vi "NMRvme3.vi"() -> ()   [LabVIEW 2013]
uses:
  <vilib>/Utility/file.llb/Read From Spreadsheet File (DBL).vi
  <vilib>/Analysis/NI_AALBase.lvlib
panel:
  in  "RemovePed":bool=TRUE
  in  "IF / LOG Det":bool
  in  "Q curve file":string="realback213.txt"
  out "File name 2":string="C:\\users\\plm\\Desktop\\rssmt\\realback213.txt"
  in  "AutoBaseline":bool
  out "RF OK":bool=TRUE
  out "Peak area (V-MHz)":sgl=0.007902089 format="%.3f"
  in  "Gauss Fit":bool
  out "NMR Graph + Fit":cluster{cluster{dbl, "Numeric":dbl}[]}[](graph)=[{[{224.37, "Numeric"=0.011213333333333334}, {224.372, "Numeric"=0.009013333333333333}, {224.374, "Numeric"=0.006013333333333334}, {224.376, "Numeric"=0.005013333333333333}, {224.37800000000001, "Numeric"=0.0029133333333333333}, {224.38, "Numeric"=-0.002886666666666667}, {224.382, "Numeric"=0.0015133333333333331}, {224.38400000000001, "Numeric"=0.006213333333333333}, {224.386, "Numeric"=-0.000986666666666667}, {224.388, "Numeric"=-0.009586666666666667}, {224.39000000000001, "Numeric"=-0.007886666666666667}, {224.392, "Numeric"=-0.0054866666666666675}, {224.394, "Numeric"=-0.011186666666666666}, {224.39600000000002, "Numeric"=-0.005086666666666666}, {224.398, "Numeric"=0.003413333333333333}, {224.4, "Numeric"=-0.006986666666666667}, {224.40200000000002, "Numeric"=-0.013286666666666667}, {224.404, "Numeric"=-0.003986666666666667}, {224.406, "Numeric"=0.003513333333333333}, {224.40800000000002, "Numeric"=-0.010286666666666666}, {224.41, "Numeric"=-0.012286666666666666}, {224.412, "Numeric"=-0.002686666666666667}, {224.41400000000002, "Numeric"=-0.0074866666666666675}, {224.416, "Numeric"=-0.013786666666666666}, {224.418, "Numeric"=-0.008786666666666667}, {224.42000000000002, "Numeric"=-0.001286666666666667}, {224.422, "Numeric"=-0.004586666666666667}, {224.424, "Numeric"=-0.013886666666666667}, {224.426, "Numeric"=-0.007186666666666668}, {224.428, "Numeric"=-0.001986666666666667}, {224.43, "Numeric"=-0.006186666666666667}, {224.432, "Numeric"=-0.002586666666666667}, {224.434, "Numeric"=0.006213333333333333}, {224.436, "Numeric"=0.006313333333333334}, {224.438, "Numeric"=0.003913333333333333}, {224.44, "Numeric"=0.009913333333333333}, {224.442, "Numeric"=0.020313333333333333}, {224.444, "Numeric"=0.018113333333333332}, {224.446, "Numeric"=0.02461333333333333}, {224.448, "Numeric"=0.038213333333333335}, {224.45, "Numeric"=0.048113333333333334}, {224.452, "Numeric"=0.059713333333333334}, {224.454, "Numeric"=0.07631333333333333}, {224.456, "Numeric"=0.11191333333333334}, {224.458, "Numeric"=0.14051333333333332}, {224.46, "Numeric"=0.17031333333333334}, {224.462, "Numeric"=0.22211333333333333}, {224.464, "Numeric"=0.2830133333333333}, {224.466, "Numeric"=0.3263133333333333}, {224.468, "Numeric"=0.3479133333333333}, {224.47, "Numeric"=0.36471333333333333}, {224.472, "Numeric"=0.3424133333333333}, {224.474, "Numeric"=0.2951133333333333}, {224.476, "Numeric"=0.23841333333333334}, {224.478, "Numeric"=0.20081333333333334}, {224.48, "Numeric"=0.16211333333333333}, {224.482, "Numeric"=0.12461333333333333}, {224.484, "Numeric"=0.09951333333333333}, {224.486, "Numeric"=0.09201333333333334}, {224.488, "Numeric"=0.07011333333333333}, {224.49, "Numeric"=0.05211333333333334}, {224.492, "Numeric"=0.04461333333333334}, {224.494, "Numeric"=0.04271333333333333}, {224.496, "Numeric"=0.02851333333333333}, {224.498, "Numeric"=0.020213333333333333}, {224.5, "Numeric"=0.023113333333333333}, {224.502, "Numeric"=0.02411333333333333}, {224.504, "Numeric"=0.009413333333333334}, {224.506, "Numeric"=0.010313333333333334}, {224.508, "Numeric"=0.016413333333333332}, {224.51, "Numeric"=0.007913333333333333}, {224.512, "Numeric"=-0.005086666666666666}, {224.514, "Numeric"=-0.001386666666666667}, {224.516, "Numeric"=0.008913333333333334}, {224.518, "Numeric"=0.006013333333333334}, {224.51999999999998, "Numeric"=-0.00048666666666666693}, {224.522, "Numeric"=-0.000986666666666667}, {224.524, "Numeric"=0.0006133333333333329}, {224.52599999999998, "Numeric"=-0.001286666666666667}, {224.528, "Numeric"=0.001813333333333333}, {224.53, "Numeric"=0.011613333333333333}, {224.53199999999998, "Numeric"=0.002213333333333333}, {224.534, "Numeric"=-0.002686666666666667}, {224.536, "Numeric"=0.006913333333333334}, {224.53799999999998, "Numeric"=0.005213333333333334}, {224.54, "Numeric"=-8.666666666666718e-05}, {224.542, "Numeric"=-0.000186666666666667}, {224.54399999999998, "Numeric"=0.0017133333333333328}, {224.546, "Numeric"=0.0026133333333333334}, {224.548, "Numeric"=-0.002786666666666667}, {224.54999999999998, "Numeric"=0.004013333333333332}, {224.552, "Numeric"=0.016813333333333333}, {224.554, "Numeric"=0.004113333333333333}, {224.55599999999998, "Numeric"=-0.003086666666666667}, {224.558, "Numeric"=0.004413333333333333}, {224.56, "Numeric"=0.011913333333333333}, {224.56199999999998, "Numeric"=0.004713333333333333}, {224.564, "Numeric"=0.0029133333333333333}, {224.566, "Numeric"=0.012713333333333333}, {224.56799999999998, "Numeric"=0.011013333333333333}, {224.57, "Numeric"=0.0006133333333333329}]}]
  in  "Amp of Q curve":dbl=1.7999999999999998 min=0.0 max=3.0 step=0.01 format="%_3f"
  in  "Subtract Q curve":bool
  in  "Adjust Tune":bool
  out "Ped Offset":dbl(graph)=0.002486666666666667
  out "Pedestal Difference":dbl(graph)=0.006853333333333334
  out "# Good Spectra":i32=49
  in  "Quality cuts":bool=TRUE
  out "Pedestal OK":bool=TRUE
  out "Sweep #":i32=5
  out "1st Sweep":bool
  out "ADC volts OK":bool=TRUE
  out "Peak Height Distribution":cluster{"Y":dbl[], "Y":dbl[]}[](graph)=[{"Y"=[0.003398266666666667, 0.0034614666666666666, 0.0035246666666666664, 0.0035878666666666666, 0.0036510666666666664, 0.0037142666666666667, 0.0037774666666666665, 0.0038406666666666663, 0.0039038666666666665, 0.003967066666666666, 0.0040302666666666665, 0.004093466666666666, 0.004156666666666666, 0.004219866666666666, 0.004283066666666666, 0.004346266666666666, 0.004409466666666666, 0.004472666666666666, 0.004535866666666666, 0.004599066666666666, 0.004662266666666666, 0.004725466666666666, 0.004788666666666666, 0.004851866666666666, 0.0049150666666666655, 0.004978266666666666, 0.005041466666666666, 0.005104666666666665, 0.005167866666666666, 0.005231066666666666, 0.005294266666666665, 0.005357466666666665, 0.005420666666666666, 0.005483866666666665, 0.005547066666666665, 0.0056102666666666655, 0.005673466666666666, 0.005736666666666665, 0.005799866666666665, 0.0058630666666666656, 0.005926266666666665, 0.005989466666666665, 0.006052666666666665, 0.006115866666666665, 0.006179066666666665, 0.006242266666666665, 0.006305466666666665, 0.006368666666666665, 0.006431866666666665, 0.0064950666666666644, 0.006558266666666665, 0.006621466666666665, 0.006684666666666664, 0.0067478666666666645, 0.006811066666666665, 0.006874266666666665, 0.006937466666666664, 0.007000666666666665, 0.007063866666666665, 0.007127066666666664, 0.007190266666666664, 0.007253466666666665, 0.007316666666666664, 0.007379866666666664, 0.0074430666666666645, 0.007506266666666664, 0.007569466666666664, 0.007632666666666664, 0.007695866666666664, 0.007759066666666664, 0.007822266666666664, 0.007885466666666664, 0.007948666666666665, 0.008011866666666664, 0.008075066666666663, 0.008138266666666664, 0.008201466666666664, 0.008264666666666663, 0.008327866666666664, 0.008391066666666664, 0.008454266666666663, 0.008517466666666664, 0.008580666666666664, 0.008643866666666663, 0.008707066666666664, 0.008770266666666663, 0.008833466666666663, 0.008896666666666664, 0.008959866666666663, 0.009023066666666663, 0.009086266666666664, 0.009149466666666663, 0.009212666666666662, 0.009275866666666664, 0.009339066666666663, 0.009402266666666662, 0.009465466666666663, 0.009528666666666663, 0.009591866666666662, 0.009655066666666663], "Y"=[1.0, 0.0, 0.0, 0.0, 0.0, 0.0, 0.0, 0.0, 0.0, 1.0, 0.0, 2.0, 0.0, 1.0, 0.0, 0.0, 2.0, 0.0, 0.0, 0.0, 3.0, 2.0, 2.0, 1.0, 2.0, 0.0, 2.0, 0.0, 0.0, 2.0, 0.0, 0.0, 1.0, 1.0, 0.0, 0.0, 0.0, 0.0, 0.0, 0.0, 1.0, 1.0, 0.0, 1.0, 1.0, 0.0, 2.0, 0.0, 0.0, 0.0, 0.0, 0.0, 0.0, 0.0, 1.0, 1.0, 1.0, 0.0, 1.0, 0.0, 1.0, 0.0, 0.0, 0.0, 0.0, 0.0, 1.0, 2.0, 0.0, 2.0, 0.0, 0.0, 0.0, 0.0, 0.0, 0.0, 1.0, 1.0, 1.0, 0.0, 0.0, 0.0, 2.0, 0.0, 0.0, 1.0, 0.0, 0.0, 1.0, 0.0, 1.0, 1.0, 0.0, 0.0, 0.0, 0.0, 0.0, 0.0, 0.0, 1.0]}]
  in  "# of Sweeps":i32=50
  out "Std Dev (V)":dbl=0.001709574673437506 format="%_2g"
  out "Peak mean (V)":dbl=0.006236360544217688 format="%_4g"
  out "Peak Height":dbl(graph)=0.36471333333333333
  in  "Raw Data":bool=TRUE
  in  "Tank RF ON":bool=TRUE
  in  "IF Atten (dB)":i8 min=0 max=35 step=5
  in  "IFoffset (V)":dbl=-1.3469355999999992 min=-5.0 max=5.0 step=0.001 format="%.4f"
  in  "Tune  (V)":dbl=1.0946000000000007 min=0.0 max=5.0 step=0.001 format="%.4f"
  in  "Hi / Lo IF Gain":bool
  out "Voltage Array":sgl[](array[numeric])=[0.0137, 0.0115, 0.0085, 0.0075, 0.0054, -0.0004, 0.004, 0.0087, 0.0015, -0.0071, -0.0054, -0.003, -0.0087, -0.0026, 0.0059, -0.0045, -0.0108, -0.0015, 0.006, -0.0078, -0.0098, -0.0002, -0.005, -0.0113, -0.0063, 0.0012, -0.0021, -0.0114, -0.0047, 0.0005, -0.0037, -0.0001, 0.0087, 0.0088, 0.0064, 0.0124, 0.0228, 0.0206, 0.0271, 0.0407, 0.0506, 0.0622, 0.0788, 0.1144, 0.143, 0.1728, 0.2246, 0.2855, 0.3288, 0.3504, 0.3672, 0.3449, 0.2976, 0.2409, 0.2033, 0.1646, 0.1271, 0.102, 0.0945, 0.0726, 0.0546, 0.0471, 0.0452, 0.031, 0.0227, 0.0256, 0.0266, 0.0119, 0.0128, 0.0189, 0.0104, -0.0026, 0.0011, 0.0114, 0.0085, 0.002, 0.0015, 0.0031, 0.0012, 0.0043, 0.0141, 0.0047, -0.0002, 0.0094, 0.0077, 0.0024, 0.0023, 0.0042, 0.0051, -0.0003, 0.0065, 0.0193, 0.0066, -0.0006, 0.0069, 0.0144, 0.0072, 0.0054, 0.0152, 0.0135, 0.0031] format="%.4f"
  in  "Invert Polarity":bool
  out "Pedestal Diff (V)":sgl=0.006853333 format="%.3f"
  out "Peak amp (V)":sgl=0.36471334 format="%.3f"
  in  "Save Data to File":bool
  in  "RF Level (dBm)":dbl=-1.0 min=-10.0 max=1.0 step=0.1 format="%.2f"
  out "SMT error out":errorcluster
  out "Sample RMS (V)":dbl=0.01349207920792079 format="%.4f"
  in  "# Sample/step":i32=100 min=1 max=1000 step=100
  in  "ADC Rate (Hz)":i32=10000 min=1 max=20000 step=1000
  in  "ADC Range":i32(ring)=1 items=["+- 10 V"=1, "+- 2.5 V"=3]
  in  "Step Width (MHz)":dbl=0.002 min=0.0 max=1000.0 step=0.0005 format="%.4f"
  in  "Freq Span (MHz)":dbl=0.2 min=0.0 max=3000.0 step=0.1 format="%.3f"
  in  "Center Freq (MHz)":dbl=224.47 min=0.005 max=6000.0 step=0.1 format="%.3f"
  in  "Sweep Mode":u16(ring)=3 items=["Off", "Single", "Auto", "Step"]
  in  "GPIB Addr (28)":refnum<visa-resource-name>="GPIB0::28::INSTR"
  # "Settings"
  # "E1039 Prototype NMR Control Panel"
  # "D\nA\nC"
  # "R\nF\n\nG\ne\nn\ne\nr\na\nt\no\nr"
  # "A\nD\nC"
  # "D\na\nt\na"
  # "I\n/\nO"
  # "Results"
  # "A\nv\ne\nr\na\ng\ne"
  # "S\nw\ne\ne\np"
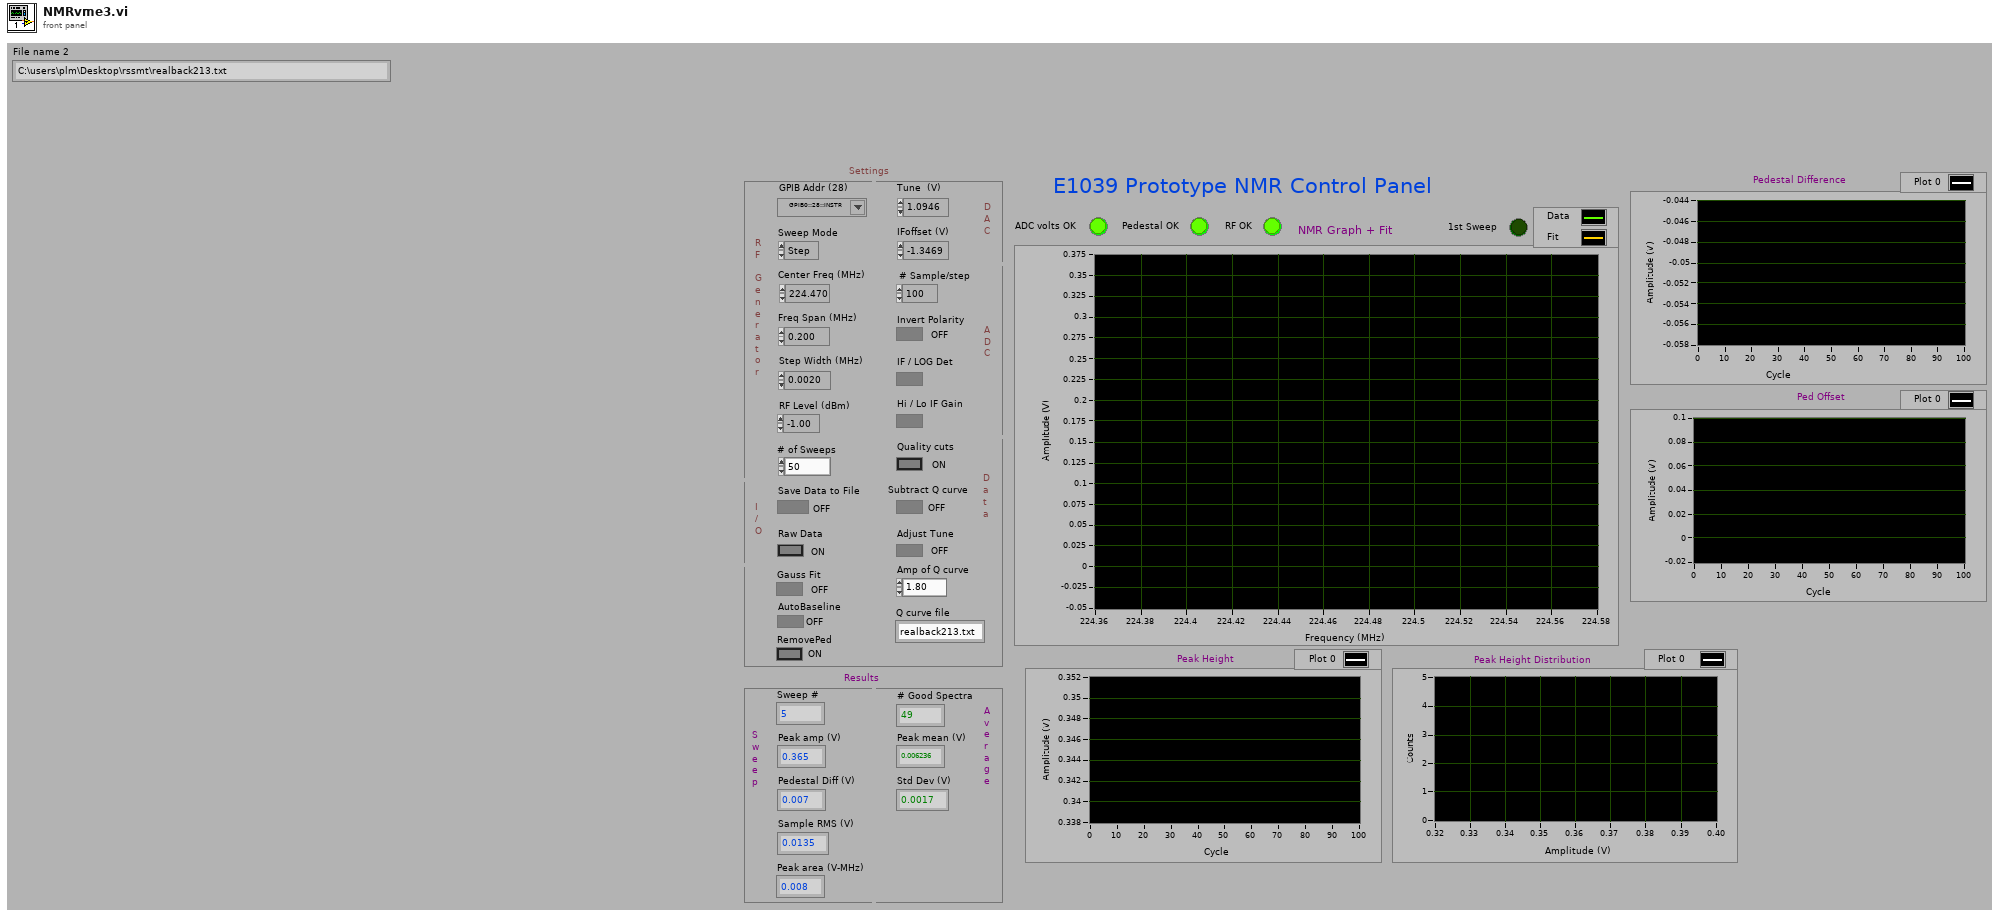
[diagram p1: front panel]
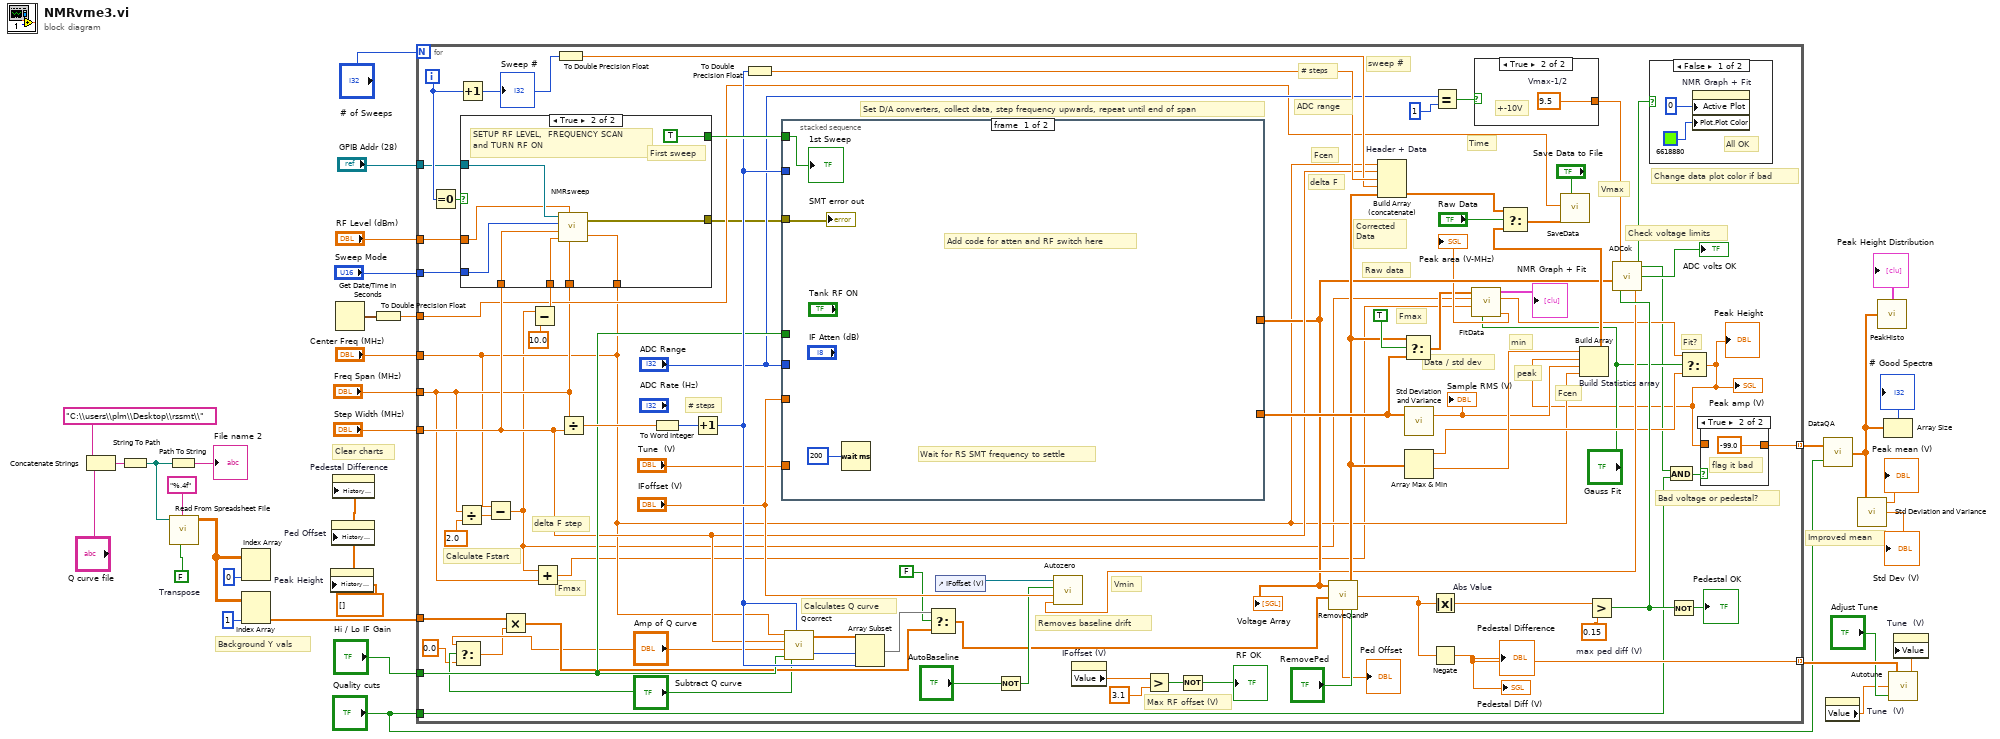
[diagram p0: block diagram]
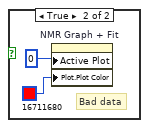
[diagram p2: hidden frame]
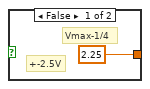
[diagram p3: hidden frame]
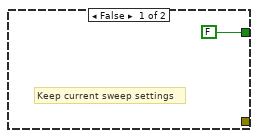
[diagram p5: hidden frame]
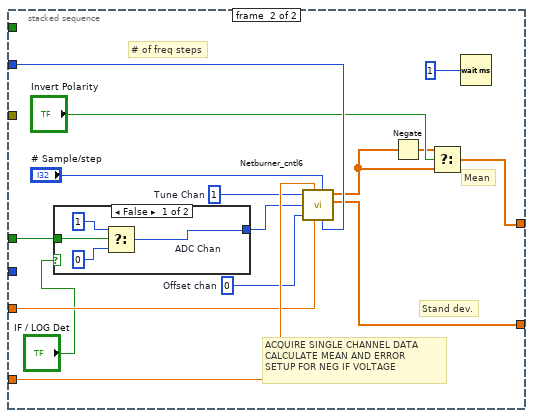
[diagram p6: hidden frame]
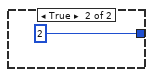
[diagram p7: hidden frame]
diagram:
  w8 = FALSE  # Transpose
  w17 = dbl[] []
  # "Background Y vals"
  # "Clear charts"
  # "Improved mean"
  n1 = Concatenate Strings "Concatenate Strings"("C:\\users\\plm\\Desktop\\rssmt\\", "Q curve file") -> (w11:string)
  n2 = String To Path(string=w11) -> (path=w7:path)
  n3 = Path To String(path=w7) -> (string=→"File name 2":string)
  n4 = call-poly <vilib>:"Read From Spreadsheet File.vi"("transpose (no:F)"=w8, "format (%.3f)"="%.4f", "file path (dialog if empty)"=w7) -> ("all rows"=w6:dbl[][])  [unwired: 4 in, 4 out]
  n5 = Index Array "Index Array"(array=w6, index (col)=0) -> ()  [unwired: 1 in, 1 out]
  n6 = Index Array(array=w6, index (col)=1) -> (element=w1:dbl[])  [unwired: 1 in]
  n7 = property on="Peak Height" class="WFChart (strict)"("History Data"=w17) -> ()  [unwired: 2 in, 2 out]
  n8 = property on="Ped Offset" class="WFChart (strict)"("History Data"=w17) -> ()  [unwired: 2 in, 2 out]
  n9 = property on="Pedestal Difference" class="WFChart (strict)"("History Data"=w17) -> ()  [unwired: 2 in, 2 out]
  n10 = Get Date/Time In Seconds() -> (seconds since 1Jan1904=w13:timestamp)
  n11 = To Double Precision Float(number=w13) -> (double precision float=w12:dbl)
  n12 = for {
    N: "# of Sweeps" -> [_]
    tunnel: [w97] -> w29 mode=indexing
    tunnel: "Quality cuts" -> [w71]
    tunnel: [w80] -> w26 mode=indexing
    tunnel: "Center Freq (MHz)" -> [w58]
    tunnel: "Freq Span (MHz)" -> [w64]
    tunnel: "Step Width (MHz)" -> [w70]
    tunnel: "Sweep Mode" -> [w84]
    tunnel: "Hi / Lo IF Gain" -> [w83]
    tunnel: "GPIB Addr (28)" -> [w82]
    tunnel: "RF Level (dBm)" -> [w81]
    tunnel: w12 -> [w65]
    tunnel: w1 -> [w43]
    i -> [w95]
    w98 = 0.15  # max ped diff (V)
    # "Vmax"
    # "Change data plot color if bad"
    # "Max RF offset (V)"
    # "Fmax"
    # "Fit?"
    # "Fmax"
    # "Time"
    # "Vmin"
    # "min"
    # "peak"
    # "Raw data"
    # "Corrected\nData"
    # "Fcen"
    # "delta F"
    # "# steps"
    # "ADC range"
    # "sweep #"
    # "Fcen"
    # "Set D/A converters, collect data, step frequency upwards, repeat until end of span"
    # "Calculates Q curve"
    # "Removes baseline drift"
    # "Bad voltage or pedestal?"
    # "Check voltage limits"
    # "Data / std dev"
    # "# steps"
    # "Calculate Fstart"
    # "delta F step"
    n13 = Equal To 0?(x=w95) -> (x = 0?=w100:bool)
    n14 = Select(t="Amp of Q curve", s="Subtract Q curve", f=0.0) -> (s? t:f=w38:dbl)
    n15 = Divide(x=w64, y=sgl 2.0) -> (x/y=w111:dbl)
    n16 = Increment(x=w95) -> (x+1=w85:i32)
    "Sweep #" <- w85
    n17 = Subtract(x=w58, y=w111) -> (x-y=w53:dbl)
    n18 = Multiply(x=w43, y=w38) -> (x*y=w42:dbl[])
    n19 = Subtract(x=w53, y=10.0) -> (x-y=w109:dbl)
    n20 = case shown="True" w100 {
      tunnel: w109 -> [_ w131]
      tunnel: w70 -> [_ w129]
      tunnel: w58 -> [_ w128]
      tunnel: w64 -> [_ w130]
      tunnel: [FALSE TRUE] -> w99
      tunnel: w84 -> [_ w126]
      tunnel: w82 -> [_ w125]
      tunnel: w81 -> [_ w124]
      tunnel: [_ w123] -> w34
      frame False {
        # "Keep current sweep settings"
      }
      frame True {
        # "First sweep"
        # "SETUP RF LEVEL,  FREQUENCY SCAN\nand TURN RF ON"
        n21 = call "NMRsweep.vi"("Center Freq (MHz)"=w128, "Freq Span (MHz)"=w130, "RF Level (dBm)"=w124, "Foffset (MHz)"=w131, "Step Width (MHz)"=w129, "Sweep Mode"=w126, "GPIB Addr (28)"=w125) -> ("error out"=w123:errorcluster)
      }
    }
    n22 = Add(x=w53, y=w64) -> (x+y=w52:dbl)
    n23 = To Double Precision Float(number=w85) -> (double precision float=w86:dbl)
    n24 = Divide(x=w64, y=w70) -> (x/y=w113:dbl)
    n25 = To Word Integer(number=w113) -> (16bit integer=w110:i16)
    n26 = Increment(x=w110) -> (x+1=w89:i16)
    n27 = To Double Precision Float(number=w89) -> (double precision float=w88:dbl)
    n28 = stacked-sequence {
      tunnel: [_ w142] -> w103
      tunnel: [_ w140] -> w68
      tunnel: w89 -> [_ w145]
      tunnel: "IFoffset (V)" -> [_ w146]
      tunnel: w83 -> [_ w137]
      tunnel: w99 -> [w133 _]
      tunnel: "ADC Range" -> [_ _]
      tunnel: "Tune  (V)" -> [_ w147]
      tunnel: w34 -> [w132 _]
      frame #0 {
        # "Add code for atten and RF switch here"
        # "Wait for RS SMT frequency to settle"
        n29 = Wait (ms)(milliseconds to wait=200) -> ()  [unwired: 1 out]
        "1st Sweep" <- w133
        "SMT error out" <- w132
      }
      frame #1 {
        w143 = 0  # Offset chan
        w144 = 1  # Tune Chan
        # "Stand dev."
        # "Mean"
        # "ACQUIRE SINGLE CHANNEL DATA\nCALCULATE MEAN AND ERROR\nSETUP FOR NEG IF VOLTAGE"
        # "# of freq steps"
        n30 = case shown="False" "IF / LOG Det" {
          tunnel: w137 -> [w153 _]
          tunnel: [w150 2] -> w136
          frame False {
            n31 = Select "ADC Chan"(t=1, s=w153, f=0) -> (s? t:f=w150:i32)
          }
          frame True {
          }
        }
        n32 = call "Netburner_cntl6.vi"("Tune DAC"=w144, "Tune Volt"=w147, "NMR ADC"=w136, "Offset DAC"=w143, "Offset Volt"=w146, "# Data"="# Sample/step", "# f steps"=w145) -> ("ADC value"=w139:dbl[], "ADC error"=w142:dbl[])  [unwired: 2 out]
        n33 = Negate(x=w139) -> (-x=w138:dbl[])
        n34 = Select(t=w138, s="Invert Polarity", f=w139) -> (s? t:f=w140:dbl[])
        n35 = Wait (ms)(milliseconds to wait=1) -> ()  [unwired: 1 out]
      }
    }
    "Voltage Array" <- w68
    n36 = call "Qcorrect.vi"("Subtract Q curve"="Subtract Q curve", "Nstep"=w89, "IF or Log"=w83, "Amp of Q curve"="Amp of Q curve", "Step Width (MHz)"=w70, "Center Freq (MHz)"=w58) -> ("Start"=w104:i32, "Array"=w105:dbl[])
    n37 = Array Subset "Array Subset"(array=w105, index=w104, length=w89) -> (w46:dbl[])
    n38 = Select(t=w46, s=FALSE, f=w42) -> (s? t:f=w45:dbl[])
    n39 = control-ref of="IFoffset (V)"() -> (w74:refnum<vi>)
    n40 = Not(x="AutoBaseline") -> (.not. x?=w47:bool)
    n41 = property on="IFoffset (V)" class="DigNum (strict)"() -> ("Value"=w62:dbl)  [unwired: 2 in, 2 out]
    n42 = Greater?(x=w62, y=3.1) -> (0:w60:bool)
    n43 = Not(x=w60) -> (.not. x?=→"RF OK":bool)
    n44 = call "RemoveQandP.vi"("Subtract Ped?"="RemovePed", "Qcurve"=w45, "Raw data"=w68) -> ("Ped L-R"=w91:dbl, "Corrected data"=w87:dbl[], "Ped Offfset"=→"Ped Offset":dbl)
    n45 = Build Array (concatenate) "Header + Data"(w58, w70, w88, w86, w87) -> (w90:dbl[])
    n46 = Select(t=w87, s=TRUE, f=w103) -> (s? t:f=w54:dbl[])
    n47 = call <vilib>:"Std Deviation and Variance.vi"("X"=w103) -> ("mean"=w69:dbl)  [unwired: 1 in, 2 out]
    "Sample RMS (V)" <- w69
    n48 = Array Max & Min(array=w87) -> (max value=w63:dbl, min value=w102:dbl)  [unwired: 2 out]
    n49 = Absolute Value "Abs Value"(x=w91) -> (abs(x)=w93:dbl)
    n50 = Negate(x=w91) -> (-x=w80:dbl)
    "Pedestal Diff (V)" <- w80
    "Pedestal Difference" <- w80
    n51 = Equal?(x="ADC Range", y=1) -> (x = y?=w78:bool)
    n52 = call "FitData.vi"("Fit?"="Gauss Fit", "Fmax"=w52, "Fmin"=w53, "Yarray"=w54) -> ("Peak Area (V-MHz)"=→"Peak area (V-MHz)":dbl, "Amplitude (V)"=w56:dbl, "NMR Graph + Fit"=→"NMR Graph + Fit":cluster{cluster{dbl, "Numeric":dbl}[]}[])  [unwired: 2 out]
    n53 = case shown="True" w78 {
      tunnel: [2.25 w119] -> w75
      frame False {
        # "Vmax-1/4"
        # "+-2.5V"
      }
      frame True {
        w119 = 9.5  # Vmax-1/2
        # "+-10V"
      }
    }
    n54 = Greater?(x=w93, y=w98) -> (0:w79:bool)
    n55 = call "ADCok.vi"("PedOK"=w79, "Array"=w68, "Vmax-1/2"=w75) -> ("Vmin"=w73:dbl, "ADC voltages OK"=→"ADC volts OK":bool, "Allok"=w50:bool)
    n56 = call "Autozero.vi"("Vmin (V)"=w73, "IFoffset (V)"="IFoffset (V)", "IF or Log"=w47, "reference"=w74) -> ()
    n57 = case shown="False" w50 {
      frame False {
        # "All OK"
        n58 = property on="NMR Graph + Fit" class="XYGraph (strict)"("Active Plot"=0, "Plot.Plot Color"=u32 6618880) -> ()  [unwired: 2 in, 2 out]
      }
      frame True {
        # "Bad data"
        n59 = property on="NMR Graph + Fit" class="XYGraph (strict)"("Active Plot"=0, "Plot.Plot Color"=u32 16711680) -> ()  [unwired: 2 in, 2 out]
      }
    }
    n60 = And(x=w50, y=w71) -> (x .and. y?=w94:bool)
    n61 = Not(x=w79) -> (.not. x?=→"Pedestal OK":bool)
    n62 = Select(t=w56, s="Gauss Fit", f=w63) -> (s? t:f=w49:dbl)
    "Peak amp (V)" <- w49
    "Peak Height" <- w49
    n63 = Build Array "Build Statistics array"(w102, w49, w69, w58) -> (w108:dbl[])
    n64 = Select(t=w90, s="Raw Data", f=w108) -> (s? t:f=w66:dbl[])
    n65 = call "SaveData.vi"("Array"=w66, "Save Data to File"="Save Data to File", "Ext time (sec)"=w65) -> ()  [unwired: 1 out]
    n66 = case shown="True" w94 {
      tunnel: [w120 -99.0] -> w97
      tunnel: w49 -> [w120 _]
      frame False {
        # "Data OK"
      }
      frame True {
        # "flag it bad"
      }
    }
  }
  n67 = call "DataQA.vi"("Quality cuts"="Quality cuts", "Data In"=w29) -> ("Data Out"=w28:dbl[])
  n68 = property on="Tune  (V)" class="DigNum (strict)"() -> ("Value"=w16:dbl)  [unwired: 2 in, 2 out]
  n69 = call <vilib>:"Std Deviation and Variance.vi"("X"=w28) -> ("mean"=→"Peak mean (V)":dbl, "standard deviation"=→"Std Dev (V)":dbl)  [unwired: 1 in, 1 out]
  n70 = call "PeakHisto.vi"("Data Out"=w28) -> ("XY Graph"=→"Peak Height Distribution":cluster{"Y":dbl[], "Y":dbl[]}[])
  n71 = Array Size(array=w28) -> (size(s)=→"# Good Spectra":i32)
  n72 = call "Autotune.vi"("Adjust Tune"="Adjust Tune", "Tune Vin"=w16, "Pedestal Diff"=w26) -> ("Tune Vout"=w15:dbl)
  n73 = property on="Tune  (V)" class="DigNum (strict)"("Value"=w15) -> ()  [unwired: 2 in, 2 out]
